vi "relativemove (SubVI).vi"(0 ".NET Refnum in":refnum<k24>, 1 "Motor Number":i32, 5 "Relative Steps":i32, 7 "Device Address In":i32, 9 "DeviceKey In":string, 11 "error in (no error)":errorcluster, 12 "stop":bool) -> (4 ".NET Refnum out":refnum<k24>, 6 "DeviceKey Out":string, 8 "Position":i32, 10 "Device Address Out":i32, 15 "error out":errorcluster)   [LabVIEW 2019]
uses:
  C:/Users/jyxks/OneDrive/Documents/Program Files/New Focus/New Focus Picomotor Application/Samples/LabVIEW/Model 8742/LabVIEW 2009/CmdLib.dll
  Program Files/New Focus/New Focus Picomotor Application/Samples/LabVIEW/Model 8742/LabVIEW 2009/CmdLib.dll
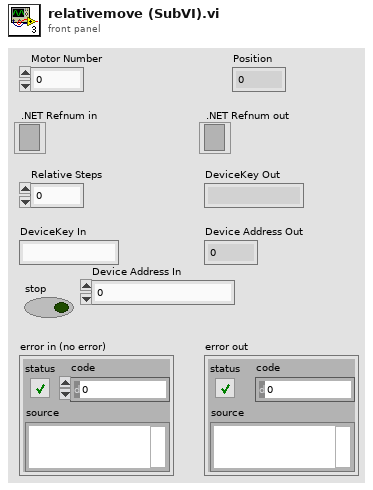
[diagram p1: front panel]
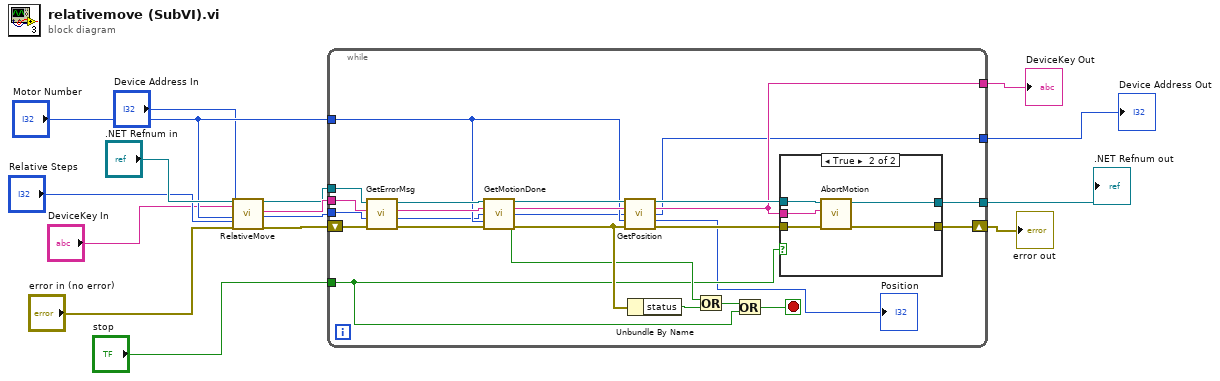
[diagram p0: block diagram]
diagram:
  n1 = call "RelativeMove.vi"("CmdLib In"=".NET Refnum in", "DeviceKey In"="DeviceKey In", "Device Address In"="Device Address In", "Motor"="Motor Number", "Relative Steps"="Relative Steps", "error in (no error)"="error in (no error)") -> ("CmdLib Out"=w9:refnum<k24>, "DeviceKey Out"=w10:string, "Device Address Out"=w14:i32, "error out"=w11:errorcluster)  [unwired: 10 in]
  n2 = while {
    tunnel: "Motor Number" -> [w36]
    tunnel: w9 -> [w35]
    tunnel: w10 -> [w34]
    tunnel: [w23] -> w6
    tunnel: w14 -> [w22]
    shift-right: [w25] -> w7
    shift-left: w11 -> [w33]
    tunnel: [w19] -> w5
    tunnel: "stop" -> [w18]
    tunnel: [w17] -> w4
    stop <- w27 stop-if-true
    n3 = call "GetErrorMsg.vi"("error in (no error)"=w33, "Device Address In"=w22, "DeviceKey In"=w34, "CmdLib In"=w35) -> ("error out"=w32:errorcluster, "Device Address Out"=w21:i32, "DeviceKey Out"=w38:string, "CmdLib Out"=w37:refnum<k24>)
    n4 = call "GetMotionDone.vi"("CmdLib In"=w37, "DeviceKey In"=w38, "Device Address In"=w21, "Motor"=w36, "error in (no error)"=w32) -> ("CmdLib Out"=w39:refnum<k24>, "DeviceKey Out"=w40:string, "Device Address Out"=w20:i32, "Is Motion Done"=w29:bool, "error out"=w30:errorcluster)  [unwired: 6 in]
    n5 = call "GetPosition.vi"("CmdLib In"=w39, "DeviceKey In"=w40, "Device Address In"=w20, "Motor"=w36, "error in (no error)"=w30) -> ("CmdLib Out"=w24:refnum<k24>, "DeviceKey Out"=w19:string, "Device Address Out"=w17:i32, "Position"=→"Position":i32, "error out"=w26:errorcluster)  [unwired: 6 in]
    n6 = Unbundle By Name(w30) -> ("status"=w31:bool)
    n7 = Or(x=w29, y=w31) -> (x .or. y?=w28:bool)
    n8 = Or(x=w28, y=w18) -> (x .or. y?=w27:bool)
    n9 = case shown="True" w18 {
      tunnel: w26 -> [w41 w47]
      tunnel: [w41 w46] -> w25
      tunnel: w24 -> [w42 w45]
      tunnel: [w42 w44] -> w23
      tunnel: w19 -> [_ w43]
      frame False {
      }
      frame True {
        n10 = call "AbortMotion.vi"("error in (no error)"=w47, "DeviceKey In"=w43, "CmdLib In"=w45) -> ("error out"=w46:errorcluster, "CmdLib Out"=w44:refnum<k24>)  [unwired: 1 in, 2 out]
      }
    }
  }
  "error out" <- w7
  ".NET Refnum out" <- w6
  "DeviceKey Out" <- w5
  "Device Address Out" <- w4
